vi "Get Lockin Status.vi"(8 "error in (no error)":errorcluster, 11 "MeasurementSMO in":refnum<class "AFM_Litho_Plugin.IV.lvclass">) -> (0 "error out":errorcluster, 2 "Status":T1=enum."created", 3 "MeasurementSMO out":refnum<class "AFM_Litho_Plugin.IV.lvclass">)   [LabVIEW 2019, in "AFM_Litho_Plugin.IV.lvclass"]
uses:
  AFM_Litho_Plugin.IV.lvclass
  Program Files (x86)/National Instruments/LabVIEW 2020/user.lib/LevyLab/Lockin-Multichannel/Instrument.DAQ/Typedefs/Get State-enum.ctl
  AFM_Litho_Plugin.IV.lvclass/AFM_Litho_Plugin.IV.ctl
  d2f37c7d-6e38-4d1d-94ab-bdb4f541719a.vi
  d2f37c7d-6e38-4d1d-94ab-bdb4f541719a.vi/ff40df25-0e41-4205-825d-56c19dc320b6.vi
  <vilib>/Utility/Debug Log/Display.vi
  <userlib>/LevyLab/Lockin-Multichannel/Instrument.Lockin/Instrument.Lockin.lvclass
  <userlib>/LevyLab/Lockin-Multichannel/Instrument.DAQ/Instrument.DAQ.lvclass
panel:
  # "Status"
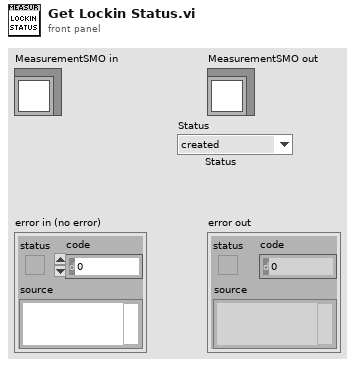
[diagram p1: front panel]
types:
  T1 = typedef "Instrument.DAQ.lvclass/Get State-enum.ctl" = enum16{"idle", "created", "started", "stopped", "sweeping"}
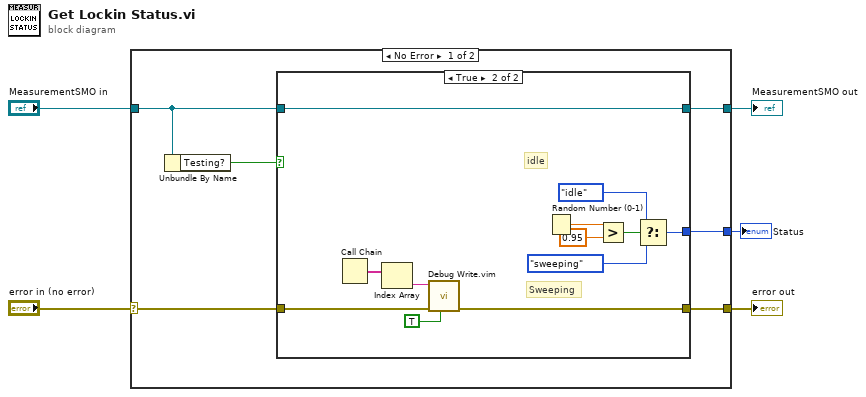
[diagram p0: block diagram]
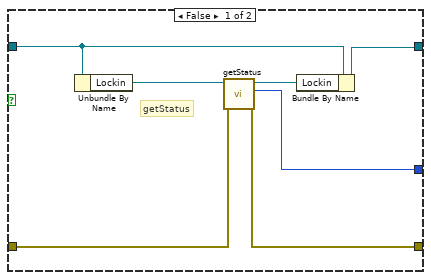
[diagram p2: hidden frame]
diagram:
  n1 = case shown="No Error" "error in (no error)" {
    selector: "error in (no error)" -> [w8 w32]
    tunnel: [w9 w32] -> w4
    tunnel: [w11 w31] -> w2
    tunnel: "MeasurementSMO in" -> [w10 w31]
    tunnel: [w6 _] -> w1
    frame No Error {
      n2 = Unbundle By Name(w10) -> ("Testing?"=w7:bool)
      n3 = case shown="True" w7 {
        tunnel: [w18 w30] -> w11
        tunnel: w10 -> [w17 w30]
        tunnel: [w13 w25] -> w9
        tunnel: w8 -> [w14 w24]
        tunnel: [w12 w26] -> w6
        frame False {
          # "getStatus"
          n4 = Unbundle By Name(w17) -> ("Lockin"=w16:refnum<class "Instrument.Lockin.lvclass">)
          n5 = call <userlib>:"getStatus.vi"("error in (no error)"=w14, "Instrument.Lockin"=w16) -> ("error out"=w13:errorcluster, "Status"=w12:T1, "Instrument.Lockin"=w15:refnum<class "Instrument.Lockin.lvclass">)  [unwired: 7 in]
          n6 = Bundle By Name(cluster=w17, "Lockin"=w15) -> (w18:refnum<class "AFM_Litho_Plugin.IV.lvclass">)
        }
        frame True {
          # "Sweeping"
          # "idle"
          n7 = Call Chain() -> (call chain=w22:string[])
          n8 = Index Array(array=w22) -> (element=w23:string)  [unwired: 1 in]
          n9 = call "Debug Write.vim"("include timestamp? (F)"=TRUE, "error in (no error)"=w24, "value"=w23) -> ("error out"=w25:errorcluster)  [unwired: 8 in]
          n10 = Random Number (0-1)() -> (number: 0 to 1=w29:dbl)
          n11 = Greater?(x=w29, y=0.95) -> (0:w27:bool)
          n12 = Select(t=Get_State-enum."idle" ("Status"), s=w27, f=Get_State-enum."sweeping" ("Status")) -> (s? t:f=w26:T1)
        }
      }
    }
    frame Error {
    }
  }
  "error out" <- w4
  "MeasurementSMO out" <- w2
  "Status" <- w1
